vi "Test Channel Control & Levels.vi"() -> ()   [LabVIEW 2020]
uses:
  VoiceMeeterRemote/Direction.ctl
  VoiceMeeterRemote/VoiceMeeterRemote/VoiceMeeterRemote.lvclass
  VoiceMeeterRemote/VoiceMeeterRemote.lvlib
panel:
  in  "Mute":bool
  out "Level":sgl(slide) scale=0.0..1.25
  in  "Gain":sgl(slide) scale=-60.0..12.0
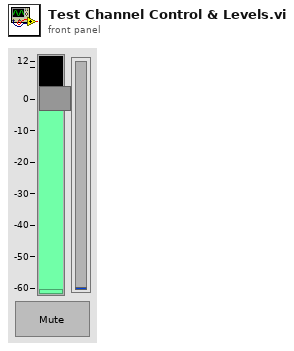
[diagram p1: front panel]
types:
  T1 = typedef "VoiceMeeterRemote.lvlib/Direction.ctl" = enum16{"Input", "Output"}
  T2 = typedef "VoiceMeeterRemote.lvlib/Levels.ctl" = cluster{"Input Pre Fader":T3[], "Input Post Fader":T3[], "Input Post Mute":T3[], "Output":T3[]}
  T3 = typedef "VoiceMeeterRemote.lvlib/Device Channels.ctl" = cluster{"Values":sgl[]}
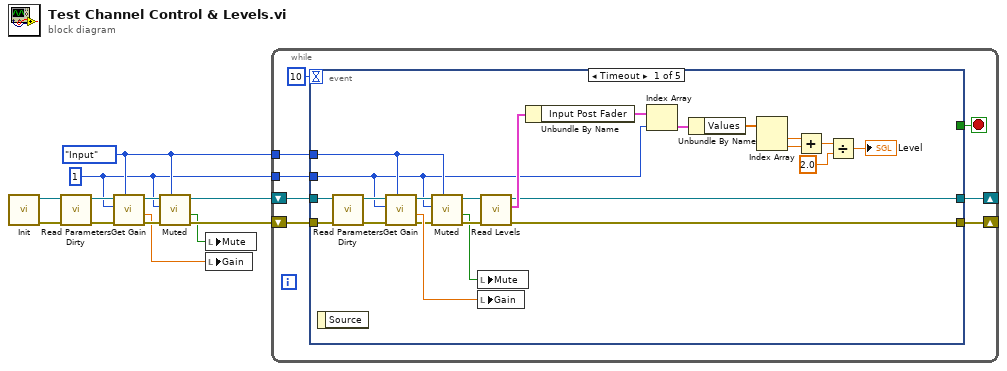
[diagram p0: block diagram]
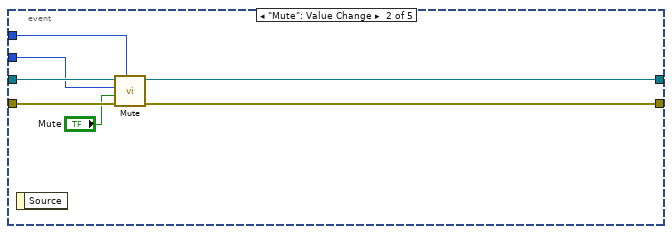
[diagram p2: hidden frame]
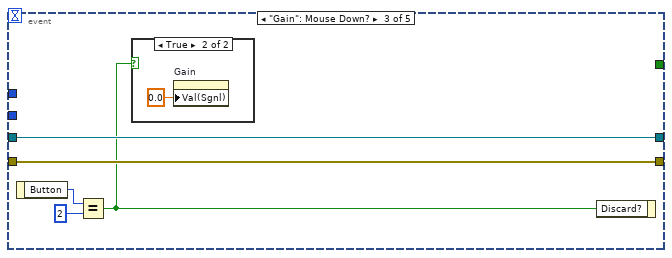
[diagram p3: hidden frame]
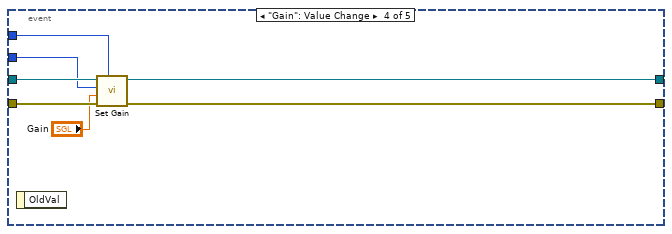
[diagram p5: hidden frame]
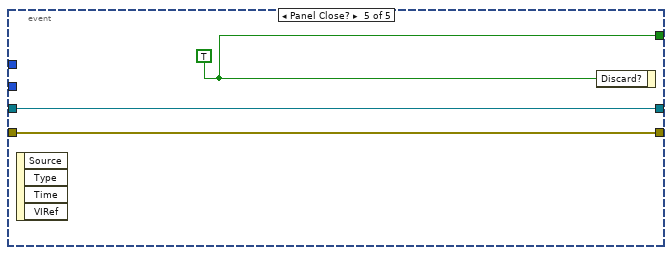
[diagram p6: hidden frame]
diagram:
  w1 = 1 ("Index")
  w2 = Direction."Input" ("Direction")
  n1 = call "Init.vi"() -> ("error out"=w11:errorcluster, "VoiceMeeterRemote out"=w12:refnum<class "VoiceMeeterRemote.lvclass">)  [unwired: 9 in, 1 out]
  n2 = call "Read Parameters Dirty.vi"("error in (no error)"=w11, "VoiceMeeterRemote in"=w12) -> ("error out"=w9:errorcluster, "VoiceMeeterRemote out"=w10:refnum<class "VoiceMeeterRemote.lvclass">)  [unwired: 7 in, 1 out]
  n3 = call "Get Gain.vi"("Direction"=w2, "error in (no error)"=w9, "Index"=w1, "VoiceMeeterRemote in"=w10) -> ("error out"=w7:errorcluster, "Value"=w3:sgl, "VoiceMeeterRemote out"=w8:refnum<class "VoiceMeeterRemote.lvclass">)  [unwired: 5 in]
  n4 = call "Muted.vi"("Direction"=w2, "error in (no error)"=w7, "Index"=w1, "VoiceMeeterRemote in"=w8) -> ("error out"=w5:errorcluster, "Muted?"=w4:bool, "VoiceMeeterRemote out"=w6:refnum<class "VoiceMeeterRemote.lvclass">)  [unwired: 5 in]
  n5 = local write "Mute"(w4) -> ()
  n6 = local write "Gain"(w3) -> ()
  n7 = while {
    shift-right: [w17] -> _
    shift-left: w6 -> [w19]
    shift-right: [w16] -> _
    shift-left: w5 -> [w18]
    tunnel: w2 -> [w14]
    tunnel: w1 -> [w13]
    stop <- w15 stop-if-true
    n8 = event shown="[0] Timeout" {
      selector: _ -> [_ _ _ _ _]
      dyn-events: _ -> [_ _ _ _ _]
      timeout: 10 -> [_ _ _ _ _]
      tunnel: w19 -> [w36 w50 w55 w63 w66]
      tunnel: w18 -> [w35 w49 w54 w62 w65]
      tunnel: [w22 w45 w55 w57 w66] -> w17
      tunnel: [w21 w44 w54 w58 w65] -> w16
      tunnel: [_ _ _ _ w64] -> w15
      tunnel: w14 -> [w32 w46 _ w61 _]
      tunnel: w13 -> [w30 w47 _ w60 _]
      event Timeout {
        n9 = event-data() -> ()  [unwired: 1 in, 1 out]
        n10 = call "Read Parameters Dirty.vi"("error in (no error)"=w35, "VoiceMeeterRemote in"=w36) -> ("error out"=w38:errorcluster, "VoiceMeeterRemote out"=w37:refnum<class "VoiceMeeterRemote.lvclass">)  [unwired: 7 in, 1 out]
        n11 = call "Get Gain.vi"("Direction"=w32, "error in (no error)"=w38, "Index"=w30, "VoiceMeeterRemote in"=w37) -> ("error out"=w40:errorcluster, "Value"=w42:sgl, "VoiceMeeterRemote out"=w39:refnum<class "VoiceMeeterRemote.lvclass">)  [unwired: 5 in]
        n12 = call "Muted.vi"("Direction"=w32, "error in (no error)"=w40, "Index"=w30, "VoiceMeeterRemote in"=w39) -> ("error out"=w43:errorcluster, "Muted?"=w41:bool, "VoiceMeeterRemote out"=w34:refnum<class "VoiceMeeterRemote.lvclass">)  [unwired: 5 in]
        n13 = local write "Mute"(w41) -> ()
        n14 = local write "Gain"(w42) -> ()
        n15 = call "Read Levels.vi"("error in (no error)"=w43, "VoiceMeeterRemote in"=w34) -> ("error out"=w21:errorcluster, "Levels"=w33:T2, "VoiceMeeterRemote out"=w22:refnum<class "VoiceMeeterRemote.lvclass">)  [unwired: 7 in]
        n16 = Unbundle By Name(w33) -> ("Input Post Fader"=w31:T3[])
        n17 = Index Array(array=w31, index=w30) -> (element=w29:T3)
        n18 = Unbundle By Name(w29) -> ("Values"=w28:sgl[])
        n19 = Index Array(array=w28) -> (element #1=w27:sgl, element #2=w26:sgl)  [unwired: 2 in]
        n20 = Add(x=w27, y=w26) -> (x+y=w25:sgl)
        n21 = Divide(x=w25, y=sgl 2.0) -> (x/y=→"Level":sgl)
      }
      event "Mute": Value Change {
        n22 = event-data() -> ()  [unwired: 1 in, 1 out]
        n23 = call "Mute.vi"("Direction"=w46, "error in (no error)"=w49, "Mute? (T)"="Mute", "Index"=w47, "VoiceMeeterRemote in"=w50) -> ("error out"=w44:errorcluster, "VoiceMeeterRemote out"=w45:refnum<class "VoiceMeeterRemote.lvclass">)  [unwired: 5 in]
      }
      event "Gain": Mouse Down? {
        n24 = event-data() -> ("Button"=w53:u16)  [unwired: 1 in]
        n25 = Equal?(x=w53, y=u16 2) -> (x = y?=w51:bool)
        n26 = case shown="True" w51 {
          frame False {
          }
          frame True {
            n27 = property on="Gain" class="Slide (strict)"("Val(Sgnl)"=sgl 0.0 ("Value (Signaling)")) -> ()  [unwired: 2 in, 2 out]
          }
        }
        n28 = event-data("Discard?"=w51) -> ()  [unwired: 1 in, 1 out]
      }
      event "Gain": Value Change {
        n29 = event-data() -> ()  [unwired: 1 in, 1 out]
        n30 = call "Set Gain.vi"("Direction"=w61, "error in (no error)"=w62, "Value"="Gain", "Index"=w60, "VoiceMeeterRemote in"=w63) -> ("error out"=w58:errorcluster, "VoiceMeeterRemote out"=w57:refnum<class "VoiceMeeterRemote.lvclass">)  [unwired: 5 in]
      }
      event Panel Close? {
        w64 = TRUE ("Discard?")
        n31 = event-data() -> ()  [unwired: 1 in, 4 out]
        n32 = event-data("Discard?"=w64) -> ()  [unwired: 1 in, 1 out]
      }
    }
  }
